vi "input.vi"(8 "error in":errorcluster, 10 "input allocation":T1, 11 "module in":refnum<class "fixed channel tag bus module.lvclass">) -> (0 "error out":errorcluster, 2 "input data":T1, 3 "module out":refnum<class "fixed channel tag bus module.lvclass">)   [LabVIEW 2013]
doc: "Provides an interface for reading data from a module at runtime. While this interface performs no operations, a child should provide an override which may read from any open sessions, references, or interfaces."
uses:
  <vilib>/NI/Tag Bus/table/data table.lvlib
  <vilib>/NI/Tag Bus/table/data polymorphs/write one/write Double.vi
  <vilib>/NI/Tag Bus/table/data table.ctl
  fixed channel tag bus module.lvclass
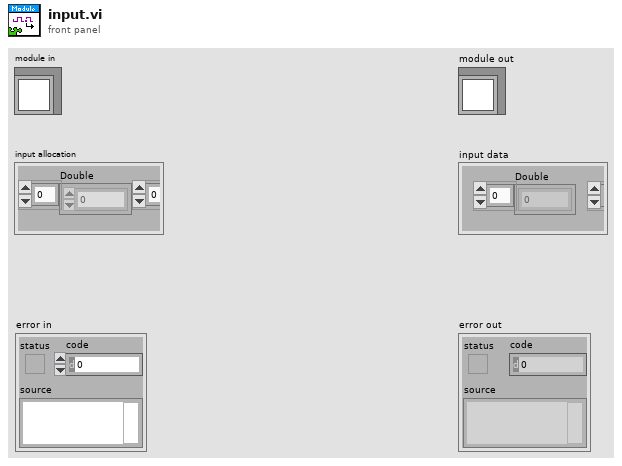
[diagram p1: front panel]
types:
  T1 = typedef "tag bus.lvlib/data table.lvlib/data table.ctl" = cluster{"Double":dbl[], "Single":sgl[], "I64":i64[], "I32":i32[], "I16":i16[], "I8":i8[], "U64":u64[], "U32":u32[], "U16":u16[], "U8":u8[], "Boolean":bool[], "String":string[], "Array of Double":cluster{"DBL Array":dbl[]}[], "Array of Single":cluster{"SGL Array":sgl[]}[], "Array of I64":cluster{"I64 Array":i64[]}[], "Array of I32":cluster{"I32 Array":i32[]}[], "Array of I16":cluster{"I16 Array":i16[]}[], "Array of I8":cluster{"I8 Array":i8[]}[], "Array of U64":cluster{"U64 Array":u64[]}[], "Array of U32":cluster{"U32 Array":u32[]}[], "Array of U16":cluster{"U16 Array":u16[]}[], "Array of U8":cluster{"U8 Array":u8[]}[], "Array of Boolean":cluster{"Boolean Array":bool[]}[], "Array of String":cluster{"String Array":string[]}[]}
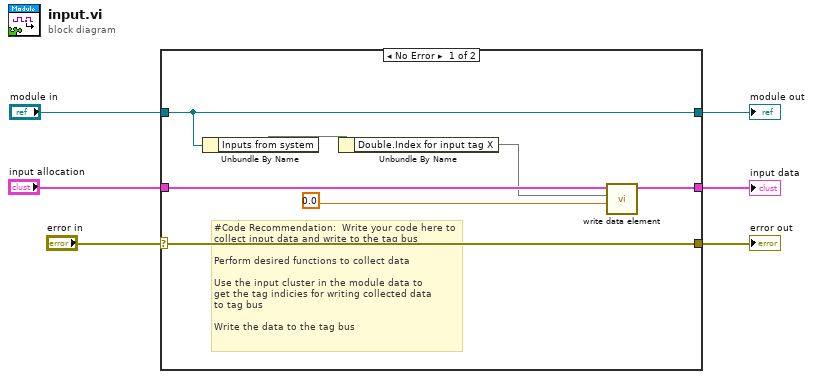
[diagram p0: block diagram]
diagram:
  n1 = case shown="No Error" "error in" {
    selector: "error in" -> [w13 w14]
    tunnel: [w13 w14] -> w5
    tunnel: [w12 w15] -> w4
    tunnel: "input allocation" -> [w11 w15]
    tunnel: "module in" -> [w10 w16]
    tunnel: [w10 w16] -> w1
    frame No Error {
      # "#Code Recommendation:  Write your code here to\ncollect input data and write to the tag bus\n\nPerform desired functions to collect data\n\nUse the input cluster in the module data to \nget the tag indicies for writing collected data\nto tag bus\n\nWrite the data to the tag bus"
      n2 = Unbundle By Name(w10) -> ("Inputs from system"=w9)
      n3 = Unbundle By Name(w9) -> ("Double.Index for input tag X"=w8)
      n4 = call-poly <vilib>:"write data element.vi"("value"=0.0, "index"=w8, "data table in"=w11) -> ("data table out"=w12:T1)  [unwired: 8 in]
    }
    frame Error {
    }
  }
  "error out" <- w5
  "module out" <- w1
  "input data" <- w4
